vi "rotate_to_wind_rel.vi"(9 "Wind Direction":dbl, 10 "Boat location":T1 {"North" format="%#_10f"; "East" format="%#_8f"}, 11 "Next Waypoint":refnum<class "Waypoint.lvclass">) -> (1 "y out":dbl, 2 "x out":dbl)   [LabVIEW 2013]
doc: "Takes in the boat location, wind angle, and waypoint location. Outputs the waypoint location in coordinates relative to boat location and rotate so wind angle is always 0."
uses:
  Data/TypeDefs/UTM Location.ctl
  Classes/Waypoint/Waypoint.lvclass
  <vilib>/Analysis/coordinate.llb/2D Cartesian Coordinate Rotation (Scalar).vi
  <vilib>/Analysis/NI_AALPro.lvlib
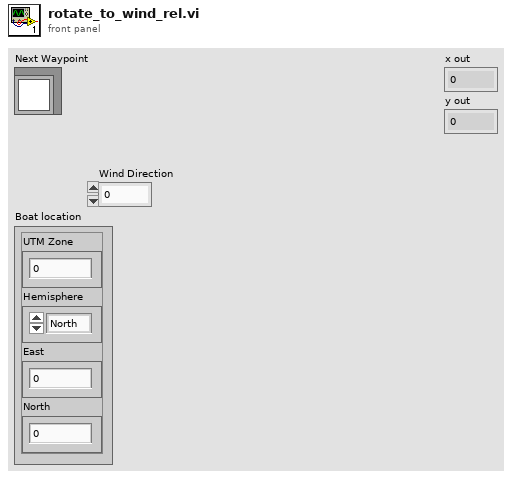
[diagram p1: front panel]
types:
  T1 = typedef "UTM Location.ctl" = cluster{"UTM Zone":dbl, "Hemisphere":enum16{"North", "South"}, "East":dbl, "North":dbl}
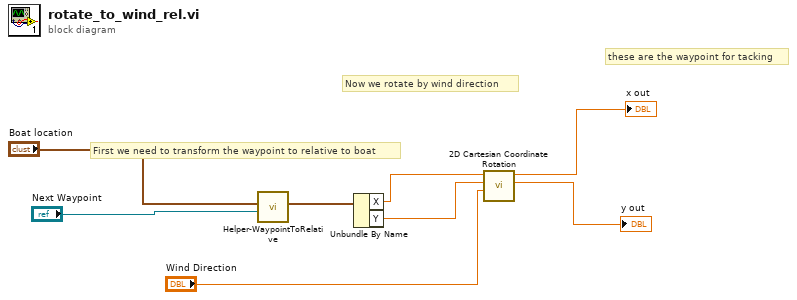
[diagram p0: block diagram]
diagram:
  # "these are the waypoint for tacking"
  # "Now we rotate by wind direction"
  # "First we need to transform the waypoint to relative to boat"
  n1 = call "Helper-WaypointToRelative.vi"("Next Waypoint"="Next Waypoint", "Boat location"="Boat location") -> ("Relative Waypoint"=w8:cluster{"X":dbl, "Y":dbl})  [unwired: 9 in]
  n2 = Unbundle By Name(w8) -> ("X"=w7:dbl, "Y"=w6:dbl)
  n3 = call-poly <vilib>:"2D Cartesian Coordinate Rotation.vi"("theta"="Wind Direction", "y"=w6, "x"=w7) -> ("y out"=→"y out":dbl, "x out"=→"x out":dbl)  [unwired: 6 in, 1 out]
